vi "FunctionGenerator.vi"(5 "Frequency (1000 Hz)":dbl=1000.0, 6 "DC Offset (0.00 V)":dbl, 7 "Waveform Function (1: Sine)":u16(ring)=1 items=["DC", "Sine", "Square", "Triangle", "Ramp", "Pulse", "Noise", "Sinc", "Negative Ramp", "Exponential Rise", "Exponential Fall", "Cardiac"], 8 "error in (no error)":errorcluster, 9 "Send settings":bool, 10 "Amplitude (1 Vpp)":dbl=1.0, 11 "VISA Refnum in":refnum<visa-resource-name>) -> (0 "error out":errorcluster, 3 "VISA Refnum out":refnum<visa-resource-name>)   [LabVIEW 2019]
uses:
  Agilent 33XXX Series/Agilent 33XXX Series.lvlib
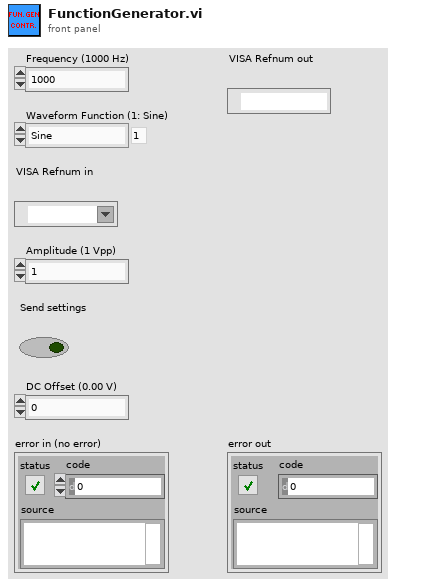
[diagram p1: front panel]
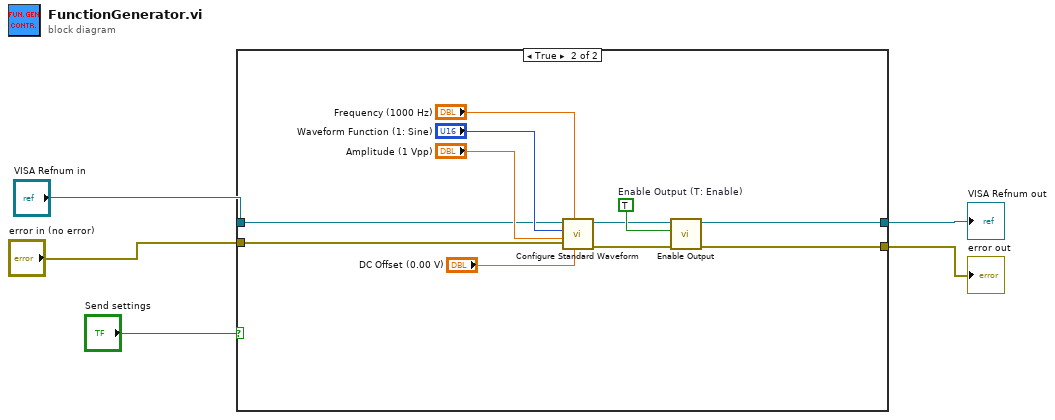
[diagram p0: block diagram]
diagram:
  n1 = case shown="True" "Send settings" {
    tunnel: "VISA Refnum in" -> [w7 w13]
    tunnel: "error in (no error)" -> [w6 w12]
    tunnel: [w6 w8] -> w3
    tunnel: [w7 w9] -> w4
    frame False {
    }
    frame True {
      w15 = TRUE  # Enable Output (T: Enable)
      n2 = call "Configure Standard Waveform.vi"("DC Offset (0.00 V)"="DC Offset (0.00 V)", "Frequency (1000 Hz)"="Frequency (1000 Hz)", "error in (no error)"=w12, "Amplitude (1)"="Amplitude (1 Vpp)", "Waveform Function (1: Sine)"="Waveform Function (1: Sine)", "VISA resource name"=w13) -> ("error out"=w10:errorcluster, "VISA resource name out"=w11:refnum<visa-resource-name>)  [unwired: 4 in]
      n3 = call "Enable Output.vi"("error in (no error)"=w10, "Enable Output  (T: Enable)"=w15, "VISA resource name"=w11) -> ("error out"=w8:errorcluster, "VISA resource name out"=w9:refnum<visa-resource-name>)  [unwired: 7 in]
    }
  }
  "VISA Refnum out" <- w4
  "error out" <- w3
